vi "Read T Controller Settings.vi"(8 "error in (no error)":errorcluster, 11 "Neocera LTC-21 in":refnum<class "Cryo-Con-22C.lvclass">) -> (0 "error out":errorcluster, 1 "Heater level":dbl, 2 "Heater mode":T1(ring), 3 "Neocera LTC-21 out":refnum<class "Cryo-Con-22C.lvclass">, 4 "PID":cluster{"P":dbl, "I":dbl, "D":dbl}, 5 "Hater range":dbl, 7 "Set point":dbl)   [LabVIEW 2015, in "Cryo-Con-22C.lvclass"]
uses:
  Cryo-Con-22C.lvclass
  Instrument/Instrument.lvclass
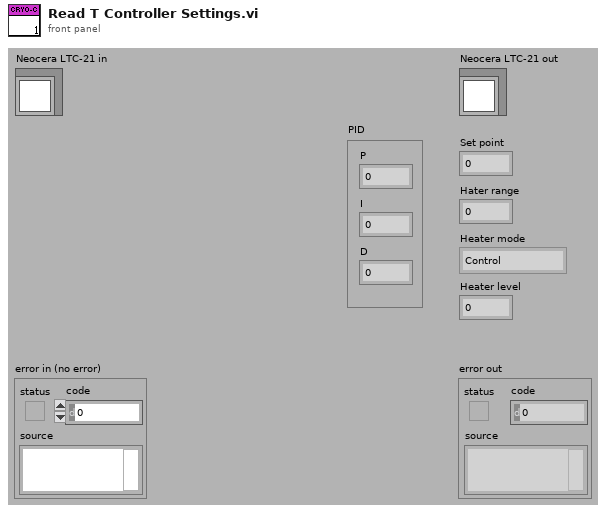
[diagram p1: front panel]
types:
  T1 = enum16{"Control", "Monitor", "Manual Heat", "Controller is in OFF mode", "Autotune is in progress"}
  T2 = enum16{"Control", "Monitor", "Manual Heat", "Controller is in OFF mode", "Autotune is in progress"}[]
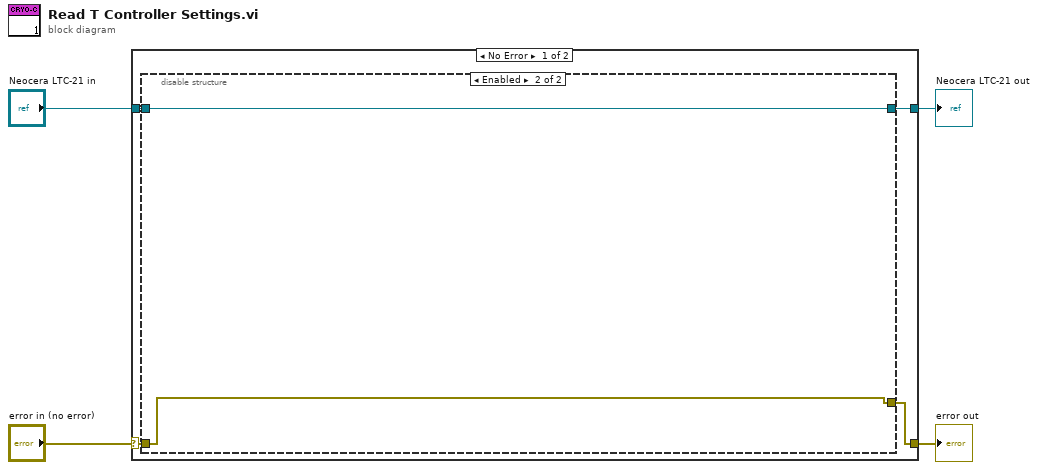
[diagram p0: block diagram]
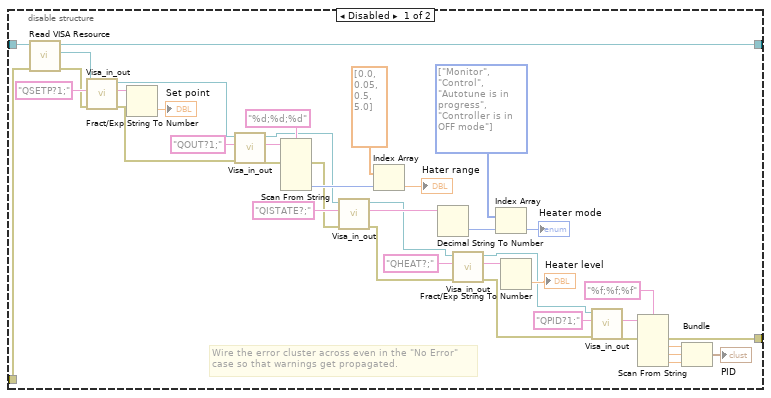
[diagram p2: hidden frame]
diagram:
  n1 = case shown="No Error" "error in (no error)" {
    selector: "error in (no error)" -> [w6 w52]
    tunnel: [w5 w52] -> w3
    tunnel: [w7 w51] -> w1
    tunnel: "Neocera LTC-21 in" -> [w8 w51]
    frame No Error {
      n2 = disable-structure shown="Enabled" {
        disable-tunnel: w8 -> [w48 w50]
        disable-tunnel: [w47 w50] -> w7
        disable-tunnel: w6 -> [w46 w49]
        disable-tunnel: [w14 w49] -> w5
        frame Disabled {
          w40 = T2 [enum."Monitor", enum."Control", enum."Autotune is in progress", enum."Controller is in OFF mode"] items=["Control", "Monitor", "Manual Heat", "Controller is in OFF mode", "Autotune is in progress"]
          # "Wire the error cluster across even in the \"No Error\"\ncase so that warnings get propagated."
          n3 = call "Read VISA Resource.vi"("error in (no error)"=w46, "Instrument.lvclass in"=w48) -> ("error out"=w20:errorcluster, "VISA Resource"=w24:refnum<visa-resource-name>, "Instrument.lvclass out"=w47:refnum<class "Cryo-Con-22C.lvclass">)  [unwired: 7 out]
          n4 = call "Visa_in_out.vi"("error in (no error)"=w20, "write buffer"="QSETP?1;", "VISA resource name"=w24) -> ("error out"=w21:errorcluster, "read buffer"=w25:string, "VISA resource name out"=w23:refnum<visa-resource-name>)  [unwired: 1 in, 5 out]
          n5 = Fract/Exp String To Number(string=w25) -> (number=→"Set point":dbl)  [unwired: 4 out]
          n6 = call "Visa_in_out.vi"("error in (no error)"=w21, "write buffer"="QOUT?1;", "VISA resource name"=w23) -> ("error out"=w29:errorcluster, "read buffer"=w33:string, "VISA resource name out"=w27:refnum<visa-resource-name>)  [unwired: 1 in, 5 out]
          n7 = Scan From String(format string="%d;%d;%d", input string=w33, error in=w29) -> (error out=w28:errorcluster, output 3=w31:i32)  [unwired: 6 in, 2 out]
          n8 = call "Visa_in_out.vi"("error in (no error)"=w28, "write buffer"="QISTATE?;", "VISA resource name"=w27) -> ("error out"=w36:errorcluster, "read buffer"=w41:string, "VISA resource name out"=w37:refnum<visa-resource-name>)  [unwired: 1 in, 5 out]
          n9 = Index Array(array=dbl[] [0.0, 0.05, 0.5, 5.0], index=w31) -> (element=→"Hater range":dbl)
          n10 = Decimal String To Number(string=w41) -> (number=w39:i32)  [unwired: 2 in, 1 out]
          n11 = call "Visa_in_out.vi"("error in (no error)"=w36, "write buffer"="QHEAT?;", "VISA resource name"=w37) -> ("error out"=w17:errorcluster, "read buffer"=w44:string, "VISA resource name out"=w9:refnum<visa-resource-name>)  [unwired: 1 in, 5 out]
          n12 = Index Array(array=w40, index=w39) -> (element=→"Heater mode":T1)
          n13 = Fract/Exp String To Number(string=w44) -> (number=→"Heater level":dbl)  [unwired: 4 out]
          n14 = call "Visa_in_out.vi"("error in (no error)"=w17, "write buffer"="QPID?1;", "VISA resource name"=w9) -> ("error out"=w15:errorcluster, "read buffer"=w18:string)  [unwired: 1 in, 6 out]
          n15 = Scan From String(format string="%f;%f;%f", input string=w18, error in=w15) -> (error out=w14:errorcluster, output 1=w13:dbl, output 2=w12:dbl, output 3=w11:dbl)  [unwired: 4 in, 2 out]
          n16 = Bundle(w13, w12, w11) -> (→"PID":cluster{dbl, dbl, dbl})  [unwired: 1 in]
        }
        frame Enabled {
        }
      }
    }
    frame Error {
    }
  }
  "error out" <- w3
  "Neocera LTC-21 out" <- w1
